vi "RichToFlatnixnet_grpc_SetPropertyRequest.vi"(5 "OutputClusterType":T1, 11 "InputCluster":T8) -> (3 "OutputCluster":T1)   [LabVIEW 2024, in "grpc-xnet_client.lvlib"]
uses:
  grpc-xnet_client.lvlib
  nixnet_grpc_SetPropertyRequest_property_id_enum/nixnet_grpc_SetPropertyRequest_property_id_enum.lvclass
  nixnet_grpc_SetPropertyRequest_property_value/nixnet_grpc_SetPropertyRequest_property_value.lvclass
  nixnet_grpc_SetPropertyRequest_property_id_enum/nixnet_grpc_SetPropertyRequest_property_id_enum.lvclass/nixnet_grpc_SetPropertyRequest_property_id_enum.ctl
  nixnet_grpc_SetPropertyRequest_property_value/nixnet_grpc_SetPropertyRequest_property_value.lvclass/nixnet_grpc_SetPropertyRequest_property_value.ctl
  nixnet_grpc_EptRxFilter_Flat.ctl
  nixnet_grpc_EptRxFilterArray_Flat.ctl
  nidevice_grpc_Session_Flat.ctl
  nixnet_grpc_DbRefArray_Flat.ctl
  nixnet_grpc_U32Array_Flat.ctl
  nixnet_grpc_Property.ctl
  nixnet_grpc_SetPropertyRequest_Flat.ctl
  nidevice_grpc_Session.ctl
  nixnet_grpc_SetPropertyRequest.ctl
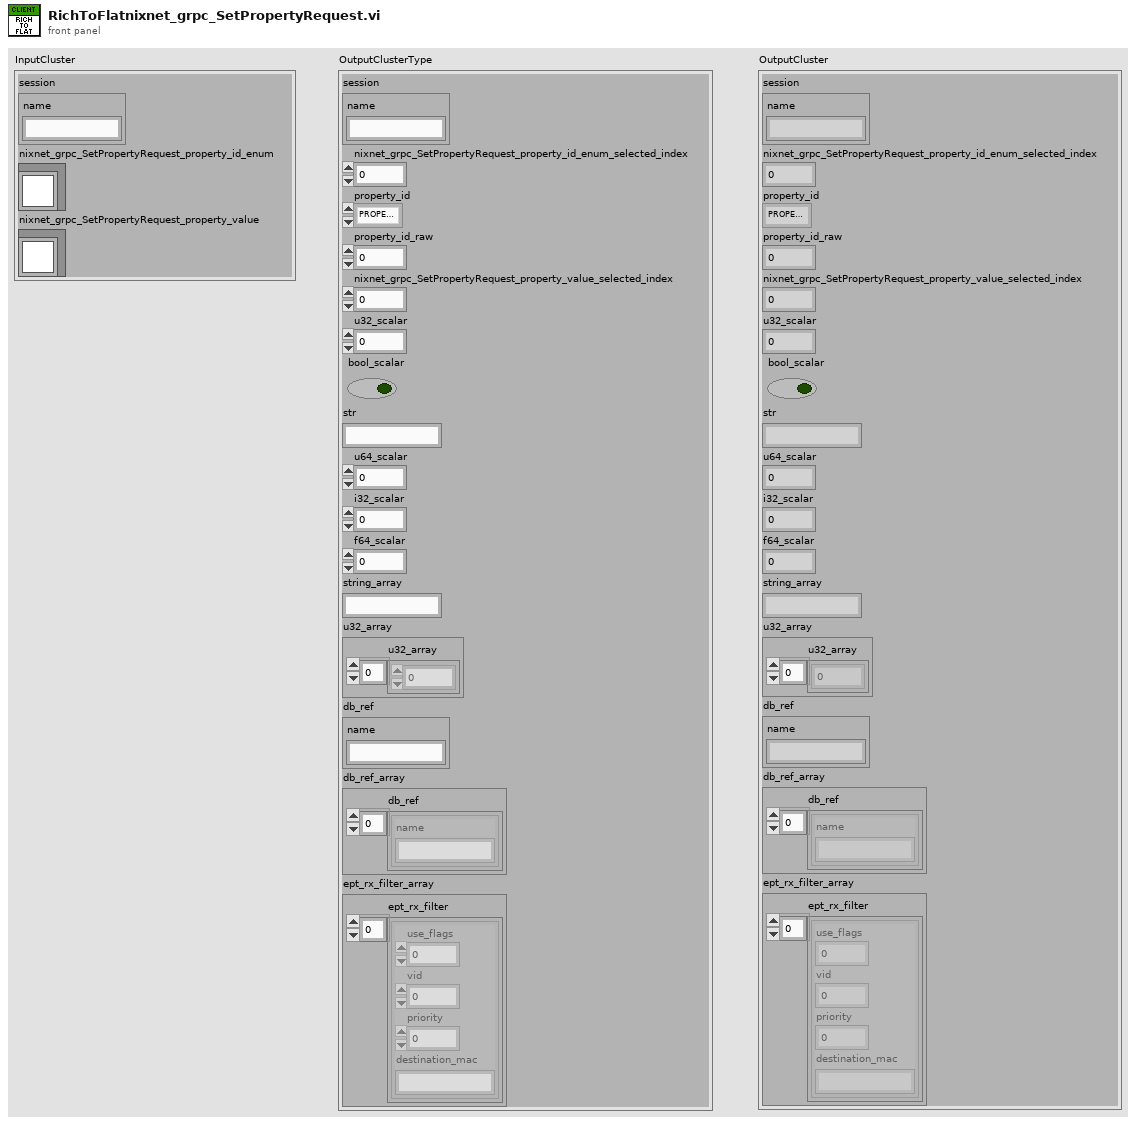
[diagram p1: front panel]
types:
  T1 = typedef "grpc-xnet_client.lvlib/nixnet_grpc_SetPropertyRequest_Flat.ctl" = cluster{"session":T2, "nixnet_grpc_SetPropertyRequest_property_id_enum_selected_index":i32, "property_id":T3, "property_id_raw":u32, "nixnet_grpc_SetPropertyRequest_property_value_selected_index":i32, "u32_scalar":u32, "bool_scalar":bool, "str":string, "u64_scalar":u64, "i32_scalar":i32, "f64_scalar":dbl, "string_array":string, "u32_array":T4, "db_ref":T2, "db_ref_array":T5, "ept_rx_filter_array":T6}
  T2 = typedef "grpc-xnet_client.lvlib/nidevice_grpc_Session_Flat.ctl" = cluster{"name":string}
  T3 = typedef "grpc-xnet_client.lvlib/nixnet_grpc_Property.ctl" = enum32{"PROPERTY_UNSPECIFIED", "PROPERTY_SESSION_APPLICATION_PROTOCOL", "PROPERTY_SESSION_AUTO_START", "PROPERTY_SESSION_CLUSTER_NAME", "PROPERTY_SESSION_DATABASE_NAME", "PROPERTY_SESSION_ENET_FRAME_FILTER", "PROPERTY_SESSION_ENET_LOG_ERROR", "PROPERTY_SESSION_ENET_LOG_FILE", "PROPERTY_SESSION_ENET_LOG_MODE", "PROPERTY_SESSION_ENET_LOG_ENABLE_MULTIPLE_FILES", "PROPERTY_SESSION_ENET_LOG_FILE_SIZE_THRESHOLD", "PROPERTY_SESSION_ENET_LOG_OPERATION", "PROPERTY_SESSION_ENET_NUM_FRAMES_RECEIVED", "PROPERTY_SESSION_ENET_SOURCE_MAC_ADDRESS_AUTO", "PROPERTY_SESSION_INTF_BAUD_RATE_64", "PROPERTY_SESSION_INTF_ADJUST_LOCAL_TIME", "PROPERTY_SESSION_INTF_BAUD_RATE", "PROPERTY_SESSION_INTF_BUS_ERR_TO_IN_STRM", "PROPERTY_SESSION_INTF_CAN_FD_BAUD_RATE_64", "PROPERTY_SESSION_INTF_CAN_DISABLE_PROT_EXCEPTION_HANDLING", "PROPERTY_SESSION_INTF_CAN_EDGE_FILTER", "PROPERTY_SESSION_INTF_CAN_EXT_TCVR_CONFIG", "PROPERTY_SESSION_INTF_CAN_FD_BAUD_RATE", "PROPERTY_SESSION_INTF_CAN_FD_ISO_MODE", "PROPERTY_SESSION_INTF_CAN_IO_MODE", "PROPERTY_SESSION_INTF_CAN_LSTN_ONLY", "PROPERTY_SESSION_INTF_CAN_PEND_TX_ORDER", "PROPERTY_SESSION_INTF_CAN_SING_SHOT", "PROPERTY_SESSION_INTF_CAN_TERM", "PROPERTY_SESSION_INTF_CAN_TCVR_STATE", "PROPERTY_SESSION_INTF_CAN_TCVR_TYPE", "PROPERTY_SESSION_INTF_CAN_TX_IO_MODE", "PROPERTY_SESSION_INTF_CAN_TRANSMIT_PAUSE", "PROPERTY_SESSION_INTF_ECHO_TX", "PROPERTY_SESSION_INTF_ENET_EPT_RECEIVE_FILTER", "PROPERTY_SESSION_INTF_ENET_EPT_TRANSMIT_BANDWIDTH", "PROPERTY_SESSION_INTF_ENET_IPV4_ADDRESS", "PROPERTY_SESSION_INTF_ENET_JUMBO_FRAMES", "PROPERTY_SESSION_INTF_ENET_LINK_SPEED", "PROPERTY_SESSION_INTF_ENET_LINK_SPEED_CONFIGURED", "PROPERTY_SESSION_INTF_ENET_MAC_ADDRESS", "PROPERTY_SESSION_INTF_ENET_OS_NETWORK_ADAPTER_DESCRIPTION", "PROPERTY_SESSION_INTF_ENET_OS_NETWORK_ADAPTER_NAME", "PROPERTY_SESSION_INTF_ENET_OPERATIONAL_STATUS", "PROPERTY_SESSION_INTF_ENET_OUT_STRM_TIMESCALE", "PROPERTY_SESSION_INTF_ENET_PHY_POWER_MODE", "PROPERTY_SESSION_INTF_ENET_PHY_STATE", "PROPERTY_SESSION_INTF_ENET_PORT_MODE", "PROPERTY_SESSION_INTF_ENET_SIGNAL_QUALITY", "PROPERTY_SESSION_INTF_ENET_SLEEP_CAPABILITY", "PROPERTY_SESSION_INTF_ENET_STATS_COUNTER_NAMES", "PROPERTY_SESSION_INTF_ENET_STATS_COUNTER_VALUES", "PROPERTY_SESSION_INTF_ENET_STATS_RX_BAD_FRAMES", "PROPERTY_SESSION_INTF_ENET_STATS_RX_BYTES", "PROPERTY_SESSION_INTF_ENET_STATS_RX_GOOD_FRAMES", "PROPERTY_SESSION_INTF_ENET_STATS_TX_BYTES", "PROPERTY_SESSION_INTF_ENET_STATS_TX_GOOD_FRAMES", "PROPERTY_SESSION_INTF_ENET_STATS_PHY_COUNTER_NAMES", "PROPERTY_SESSION_INTF_ENET_STATS_PHY_COUNTER_VALUES", "PROPERTY_SESSION_INTF_ENET_STATS_PHY_LOW_POWER_SLEEP", "PROPERTY_SESSION_INTF_ENET_STATS_PHY_SLEEP_FAILURE", "PROPERTY_SESSION_INTF_ENET_STATS_PHY_WAKEUP_FAILURE", "PROPERTY_SESSION_INTF_ENET_STATS_PHY_WAKEUP_PULSE", "PROPERTY_SESSION_INTF_ENET_STATS_PHY_WAKEUP_REQUEST", "PROPERTY_SESSION_INTF_ENET_TIME_ADJUST_NETWORK_TIME", "PROPERTY_SESSION_INTF_ENET_TIME_BMCA_ENABLED", "PROPERTY_SESSION_INTF_ENET_TIME_CLK_ACCURACY", "PROPERTY_SESSION_INTF_ENET_TIME_CLK_CLASS", "PROPERTY_SESSION_INTF_ENET_TIME_CLK_ID", "PROPERTY_SESSION_INTF_ENET_TIME_CLK_OFFSET_VAR", "PROPERTY_SESSION_INTF_ENET_TIME_GM_CLK_ACCURACY", "PROPERTY_SESSION_INTF_ENET_TIME_GM_CLK_CLASS", "PROPERTY_SESSION_INTF_ENET_TIME_GM_CLK_ID", "PROPERTY_SESSION_INTF_ENET_TIME_GM_CLK_OFFSET_VAR", "PROPERTY_SESSION_INTF_ENET_TIME_GM_PRIORITY_1", "PROPERTY_SESSION_INTF_ENET_TIME_GM_PRIORITY_2", "PROPERTY_SESSION_INTF_ENET_TIME_OFFSET_FROM_MASTER", "PROPERTY_SESSION_INTF_ENET_TIME_PORT_AS_CAPABLE", "PROPERTY_SESSION_INTF_ENET_TIME_PORT_ANNOUNCE_RECEIPT_TIMEOUT", "PROPERTY_SESSION_INTF_ENET_TIME_PORT_ANNOUNCE_TRANSMIT_ENABLED", "PROPERTY_SESSION_INTF_ENET_TIME_PORT_LOG_ANNOUNCE_INTERVAL", "PROPERTY_SESSION_INTF_ENET_TIME_PORT_LOG_ANNOUNCE_INTERVAL_CONFIGURED", "PROPERTY_SESSION_INTF_ENET_TIME_PORT_LOG_PDELAY_INTERVAL", "PROPERTY_SESSION_INTF_ENET_TIME_PORT_LOG_PDELAY_INTERVAL_CONFIGURED", "PROPERTY_SESSION_INTF_ENET_TIME_PORT_LOG_SYNC_INTERVAL", "PROPERTY_SESSION_INTF_ENET_TIME_PORT_LOG_SYNC_INTERVAL_CONFIGURED", "PROPERTY_SESSION_INTF_ENET_TIME_PORT_PDELAY_ENABLED", "PROPERTY_SESSION_INTF_ENET_TIME_PORT_STATE", "PROPERTY_SESSION_INTF_ENET_TIME_PORT_STATE_CONFIGURED", "PROPERTY_SESSION_INTF_ENET_TIME_PORT_PROP_DELAY", "PROPERTY_SESSION_INTF_ENET_TIME_PORT_PROP_DELAY_CONFIGURED", "PROPERTY_SESSION_INTF_ENET_TIME_PORT_PROP_DELAY_THRESHOLD", "PROPERTY_SESSION_INTF_ENET_TIME_PORT_STATS_COUNTER_NAMES", "PROPERTY_SESSION_INTF_ENET_TIME_PORT_STATS_COUNTER_VALUES", "PROPERTY_SESSION_INTF_ENET_TIME_PORT_STATS_RX_ANNOUNCE", "PROPERTY_SESSION_INTF_ENET_TIME_PORT_STATS_RX_PDELAY_REQUEST", "PROPERTY_SESSION_INTF_ENET_TIME_PORT_STATS_RX_SYNC", "PROPERTY_SESSION_INTF_ENET_TIME_PORT_STATS_TX_ANNOUNCE", "PROPERTY_SESSION_INTF_ENET_TIME_PORT_STATS_TX_PDELAY_REQUEST", "PROPERTY_SESSION_INTF_ENET_TIME_PORT_STATS_TX_SYNC", "PROPERTY_SESSION_INTF_ENET_TIME_PORT_SYNC_RECEIPT_TIMEOUT", "PROPERTY_SESSION_INTF_ENET_TIME_PORT_SYNC_STATUS", "PROPERTY_SESSION_INTF_ENET_TIME_PORT_SYNCED", "PROPERTY_SESSION_INTF_ENET_TIME_PRIORITY_1", "PROPERTY_SESSION_INTF_ENET_TIME_PRIORITY_2", "PROPERTY_SESSION_INTF_ENET_TIME_PROTOCOL", "PROPERTY_SESSION_INTF_ENET_TIME_PROTOCOL_ENABLED", "PROPERTY_SESSION_INTF_ENET_TIME_STEPS_TO_GM", "PROPERTY_SESSION_INTF_ENET_TRIGGER_PPS_SYNCED", "PROPERTY_SESSION_INTF_FLEX_RAY_ACC_START_RNG", "PROPERTY_SESSION_INTF_FLEX_RAY_ALW_HLT_CLK", "PROPERTY_SESSION_INTF_FLEX_RAY_ALW_PASS_ACT", "PROPERTY_SESSION_INTF_FLEX_RAY_AUTO_ASLP_WHN_STP", "PROPERTY_SESSION_INTF_FLEX_RAY_CLST_DRIFT_DMP", "PROPERTY_SESSION_INTF_FLEX_RAY_COLDSTART", "PROPERTY_SESSION_INTF_FLEX_RAY_CONNECTED_CHS", "PROPERTY_SESSION_INTF_FLEX_RAY_DEC_CORR", "PROPERTY_SESSION_INTF_FLEX_RAY_DELAY_COMP_A", "PROPERTY_SESSION_INTF_FLEX_RAY_DELAY_COMP_B", "PROPERTY_SESSION_INTF_FLEX_RAY_KEY_SLOT_ID", "PROPERTY_SESSION_INTF_FLEX_RAY_LATEST_TX", "PROPERTY_SESSION_INTF_FLEX_RAY_LIST_TIMO", "PROPERTY_SESSION_INTF_FLEX_RAY_MAC_INIT_OFF_A", "PROPERTY_SESSION_INTF_FLEX_RAY_MAC_INIT_OFF_B", "PROPERTY_SESSION_INTF_FLEX_RAY_MAX_DRIFT", "PROPERTY_SESSION_INTF_FLEX_RAY_MIC_INIT_OFF_A", "PROPERTY_SESSION_INTF_FLEX_RAY_MIC_INIT_OFF_B", "PROPERTY_SESSION_INTF_FLEX_RAY_MICROTICK", "PROPERTY_SESSION_INTF_FLEX_RAY_NULL_TO_IN_STRM", "PROPERTY_SESSION_INTF_FLEX_RAY_OFF_CORR", "PROPERTY_SESSION_INTF_FLEX_RAY_OFF_CORR_OUT", "PROPERTY_SESSION_INTF_FLEX_RAY_RATE_CORR", "PROPERTY_SESSION_INTF_FLEX_RAY_RATE_CORR_OUT", "PROPERTY_SESSION_INTF_FLEX_RAY_SAMP_PER_MICRO", "PROPERTY_SESSION_INTF_FLEX_RAY_SING_SLOT_EN", "PROPERTY_SESSION_INTF_FLEX_RAY_SLEEP", "PROPERTY_SESSION_INTF_FLEX_RAY_STATISTICS_EN", "PROPERTY_SESSION_INTF_FLEX_RAY_SYM_TO_IN_STRM", "PROPERTY_SESSION_INTF_FLEX_RAY_SYNC_STATUS", "PROPERTY_SESSION_INTF_FLEX_RAY_SYNC_CH_A_EVEN", "PROPERTY_SESSION_INTF_FLEX_RAY_SYNC_CH_A_ODD", "PROPERTY_SESSION_INTF_FLEX_RAY_SYNC_CH_B_EVEN", "PROPERTY_SESSION_INTF_FLEX_RAY_SYNC_CH_B_ODD", "PROPERTY_SESSION_INTF_FLEX_RAY_TERM", "PROPERTY_SESSION_INTF_FLEX_RAY_WAKEUP_CH", "PROPERTY_SESSION_INTF_FLEX_RAY_WAKEUP_PTRN", "PROPERTY_SESSION_INTF_NAME", "PROPERTY_SESSION_INTF_LIN_BREAK_DELIMITER_LENGTH", "PROPERTY_SESSION_INTF_LIN_BREAK_LENGTH", "PROPERTY_SESSION_INTF_LIN_CHECKSUM_TO_IN_STRM", "PROPERTY_SESSION_INTF_LIN_DIAG_P2_MIN", "PROPERTY_SESSION_INTF_LIN_DIAG_ST_MIN", "PROPERTY_SESSION_INTF_LIN_MASTER", "PROPERTY_SESSION_INTF_LIN_NO_RESPONSE_TO_IN_STRM", "PROPERTY_SESSION_INTF_LINO_STR_SLV_RSP_LST_BY_NAD", "PROPERTY_SESSION_INTF_LIN_SCHED_NAMES", "PROPERTY_SESSION_INTF_LIN_SLEEP", "PROPERTY_SESSION_INTF_LIN_ALW_START_WO_BUS_PWR", "PROPERTY_SESSION_INTF_LIN_TERM", "PROPERTY_SESSION_INTF_OUT_STRM_LIST", "PROPERTY_SESSION_INTF_OUT_STRM_LIST_BY_ID", "PROPERTY_SESSION_INTF_OUT_STRM_TIMNG", "PROPERTY_SESSION_INTF_SRC_TERM_START_TRIGGER", "PROPERTY_SESSION_INTF_START_TRIG_TO_IN_STRM", "PROPERTY_SESSION_LIST", "PROPERTY_SESSION_MODE", "PROPERTY_SESSION_NUM_IN_LIST", "PROPERTY_SESSION_NUM_FRAMES", "PROPERTY_SESSION_NUM_PEND", "PROPERTY_SESSION_NUM_UNUSED", "PROPERTY_SESSION_PAYLD_LEN_MAX", "PROPERTY_SESSION_PROTOCOL", "PROPERTY_SESSION_QUEUE_SIZE", "PROPERTY_SESSION_RESAMP_RATE", "PROPERTY_SESSION_J1939_ECU", "PROPERTY_SESSION_J1939_ECU_BUSY", "PROPERTY_SESSION_J1939_FILL_BYTE", "PROPERTY_SESSION_J1939_INCLUDE_DEST_ADDR_IN_PGN", "PROPERTY_SESSION_J1939_MAX_REPEAT_CTS", "PROPERTY_SESSION_J1939_ADDRESS", "PROPERTY_SESSION_J1939_NAME", "PROPERTY_SESSION_J1939_NUM_PACKETS_RECV", "PROPERTY_SESSION_J1939_NUM_PACKETS_RESP", "PROPERTY_SESSION_J1939_HOLD_TIME_TH", "PROPERTY_SESSION_J1939_RESPONSE_TIME_TR_GD", "PROPERTY_SESSION_J1939_RESPONSE_TIME_TR_SD", "PROPERTY_SESSION_J1939_TIMEOUT_T1", "PROPERTY_SESSION_J1939_TIMEOUT_T2", "PROPERTY_SESSION_J1939_TIMEOUT_T3", "PROPERTY_SESSION_J1939_TIMEOUT_T4", "PROPERTY_SESSION_J1939_WRITE_QUEUE_SIZE", "PROPERTY_SYS_CDAQ_PKT_TIME", "PROPERTY_SYS_DEV_REFS", "PROPERTY_SYS_INTF_REFS", "PROPERTY_SYS_INTF_REFS_ALL", "PROPERTY_SYS_INTF_REFS_CAN", "PROPERTY_SYS_INTF_REFS_ETHERNET", "PROPERTY_SYS_INTF_REFS_FLEX_RAY", "PROPERTY_SYS_INTF_REFS_LIN", "PROPERTY_SYS_VER_BUILD", "PROPERTY_SYS_VER_MAJOR", "PROPERTY_SYS_VER_MINOR", "PROPERTY_SYS_VER_PHASE", "PROPERTY_SYS_VER_UPDATE", "PROPERTY_DEV_FORM_FAC", "PROPERTY_DEV_INTF_REFS", "PROPERTY_DEV_INTF_REFS_ALL", "PROPERTY_DEV_NUM_PORTS", "PROPERTY_DEV_NUM_PORTS_ALL", "PROPERTY_DEV_NAME", "PROPERTY_DEV_PRODUCT_NUM", "PROPERTY_DEV_SER_NUM", "PROPERTY_DEV_SLOT_NUM", "PROPERTY_INTF_CAN_TERM_CAP", "PROPERTY_INTF_CAN_TCVR_CAP", "PROPERTY_INTF_DEV_REF", "PROPERTY_INTF_DONGLE_COMPATIBLE_FIRMWARE_VERSION", "PROPERTY_INTF_DONGLE_COMPATIBLE_REVISION", "PROPERTY_INTF_DONGLE_FIRMWARE_VERSION", "PROPERTY_INTF_DONGLE_ID", "PROPERTY_INTF_DONGLE_REVISION", "PROPERTY_INTF_DONGLE_STATE", "PROPERTY_INTF_NAME", "PROPERTY_INTF_NUM", "PROPERTY_INTF_PORT_NUM", "PROPERTY_INTF_PROTOCOL"}
  T4 = typedef "grpc-xnet_client.lvlib/nixnet_grpc_U32Array_Flat.ctl" = cluster{"u32_array":u32[]}
  T5 = typedef "grpc-xnet_client.lvlib/nixnet_grpc_DbRefArray_Flat.ctl" = cluster{"db_ref":T2[]}
  T6 = typedef "grpc-xnet_client.lvlib/nixnet_grpc_EptRxFilterArray_Flat.ctl" = cluster{"ept_rx_filter":T7[]}
  T7 = typedef "grpc-xnet_client.lvlib/nixnet_grpc_EptRxFilter_Flat.ctl" = cluster{"use_flags":u32, "vid":u32, "priority":u32, "destination_mac":string}
  T8 = typedef "grpc-xnet_client.lvlib/nixnet_grpc_SetPropertyRequest.ctl" = cluster{"session":T9, "nixnet_grpc_SetPropertyRequest_property_id_enum":refnum<class "nixnet_grpc_SetPropertyRequest_property_id_enum.lvclass">, "nixnet_grpc_SetPropertyRequest_property_value":refnum<class "nixnet_grpc_SetPropertyRequest_property_value.lvclass">}
  T9 = typedef "grpc-xnet_client.lvlib/nidevice_grpc_Session.ctl" = cluster{"name":string}
  T10 = typedef "grpc-xnet_client.lvlib/nixnet_grpc_U32Array.ctl" = cluster{"u32_array":u32[]}
  T11 = typedef "grpc-xnet_client.lvlib/nixnet_grpc_DbRefArray.ctl" = cluster{"db_ref":T9[]}
  T12 = typedef "grpc-xnet_client.lvlib/nixnet_grpc_EptRxFilterArray.ctl" = cluster{"ept_rx_filter":T13[]}
  T13 = typedef "grpc-xnet_client.lvlib/nixnet_grpc_EptRxFilter.ctl" = cluster{"use_flags":u32, "vid":u32, "priority":u32, "destination_mac":string}
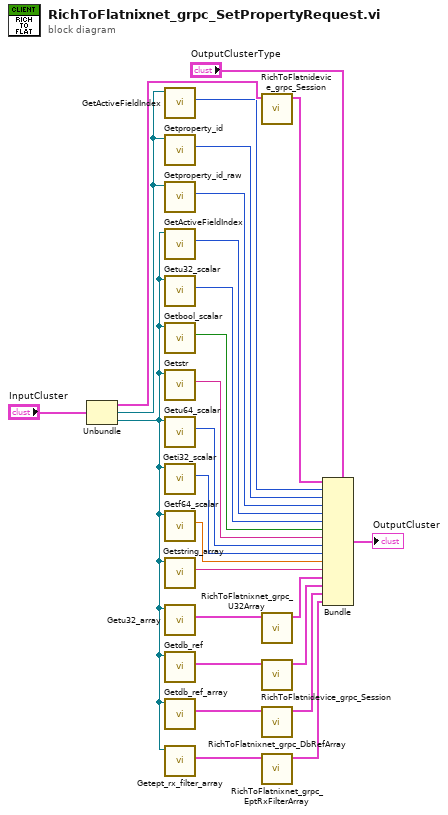
[diagram p0: block diagram]
diagram:
  n1 = Unbundle "Unbundle"("InputCluster") -> ("session"=w23:T9, "nixnet_grpc_SetPropertyRequest_property_id_enum"=w21:refnum<class "nixnet_grpc_SetPropertyRequest_property_id_enum.lvclass">, "nixnet_grpc_SetPropertyRequest_property_value"=w17:refnum<class "nixnet_grpc_SetPropertyRequest_property_value.lvclass">)
  n2 = call "GetActiveFieldIndex.vi"("OneOfTemplate in"=w21) -> ("Active Field Index"=w20:i32)  [unwired: 8 in, 2 out]
  n3 = call "Getproperty_id.vi"("OneOfTemplate in"=w21) -> ("Get_Val"=w19:T3)  [unwired: 8 in, 2 out]
  n4 = call "Getproperty_id_raw.vi"("OneOfTemplate in"=w21) -> ("Get_Val"=w18:u32)  [unwired: 8 in, 2 out]
  n5 = call "GetActiveFieldIndex.vi"("OneOfTemplate in"=w17) -> ("Active Field Index"=w16:i32)  [unwired: 8 in, 2 out]
  n6 = call "Getu32_scalar.vi"("OneOfTemplate in"=w17) -> ("Get_Val"=w15:u32)  [unwired: 8 in, 2 out]
  n7 = call "Getbool_scalar.vi"("OneOfTemplate in"=w17) -> ("Get_Val"=w14:bool)  [unwired: 8 in, 2 out]
  n8 = call "Getstr.vi"("OneOfTemplate in"=w17) -> ("Get_Val"=w13:string)  [unwired: 8 in, 2 out]
  n9 = call "Getu64_scalar.vi"("OneOfTemplate in"=w17) -> ("Get_Val"=w12:u64)  [unwired: 8 in, 2 out]
  n10 = call "Geti32_scalar.vi"("OneOfTemplate in"=w17) -> ("Get_Val"=w11:i32)  [unwired: 8 in, 2 out]
  n11 = call "Getf64_scalar.vi"("OneOfTemplate in"=w17) -> ("Get_Val"=w10:dbl)  [unwired: 8 in, 2 out]
  n12 = call "Getstring_array.vi"("OneOfTemplate in"=w17) -> ("Get_Val"=w9:string)  [unwired: 8 in, 2 out]
  n13 = call "Getu32_array.vi"("OneOfTemplate in"=w17) -> ("Get_Val"=w8:T10)  [unwired: 8 in, 2 out]
  n14 = call "Getdb_ref.vi"("OneOfTemplate in"=w17) -> ("Get_Val"=w6:T9)  [unwired: 8 in, 2 out]
  n15 = call "Getdb_ref_array.vi"("OneOfTemplate in"=w17) -> ("Get_Val"=w4:T11)  [unwired: 8 in, 2 out]
  n16 = call "Getept_rx_filter_array.vi"("OneOfTemplate in"=w17) -> ("Get_Val"=w2:T12)  [unwired: 8 in, 2 out]
  n17 = call "RichToFlatnidevice_grpc_Session.vi"("InputCluster"=w23) -> ("OutputCluster"=w22:T2)  [unwired: 10 in]
  n18 = call "RichToFlatnixnet_grpc_U32Array.vi"("InputCluster"=w8) -> ("OutputCluster"=w7:T4)  [unwired: 10 in]
  n19 = call "RichToFlatnidevice_grpc_Session.vi"("InputCluster"=w6) -> ("OutputCluster"=w5:T2)  [unwired: 10 in]
  n20 = call "RichToFlatnixnet_grpc_DbRefArray.vi"("InputCluster"=w4) -> ("OutputCluster"=w3:T5)  [unwired: 10 in]
  n21 = call "RichToFlatnixnet_grpc_EptRxFilterArray.vi"("InputCluster"=w2) -> ("OutputCluster"=w1:T6)  [unwired: 10 in]
  n22 = Bundle "Bundle"(cluster="OutputClusterType", "session"=w22, "nixnet_grpc_SetPropertyRequest_property_id_enum_selected_index"=w20, "property_id"=w19, "property_id_raw"=w18, "nixnet_grpc_SetPropertyRequest_property_value_selected_index"=w16, "u32_scalar"=w15, "bool_scalar"=w14, "str"=w13, "u64_scalar"=w12, "i32_scalar"=w11, "f64_scalar"=w10, "string_array"=w9, "u32_array"=w7, "db_ref"=w5, "db_ref_array"=w3, "ept_rx_filter_array"=w1) -> (→"OutputCluster":T1)
